vi "getProcedureList.vi"(8 "error in (no error)":errorcluster, 11 "IList in":refnum<class "IList.lvclass">) -> (0 "error out":errorcluster, 2 "devices out":refnum<class "IProcedure.lvclass">[](array[class]))   [LabVIEW 2022 SP3, in "openDAQ.lvlib" / "daqCoreTypes.lvlib" / "IList.lvclass"]
uses:
  IList.lvclass
  IProcedure/IProcedure.lvclass
  Errors/TypeDef/errorCodes.ctl
  Errors/Errors.lvclass
  IIterator/IIterator.lvclass
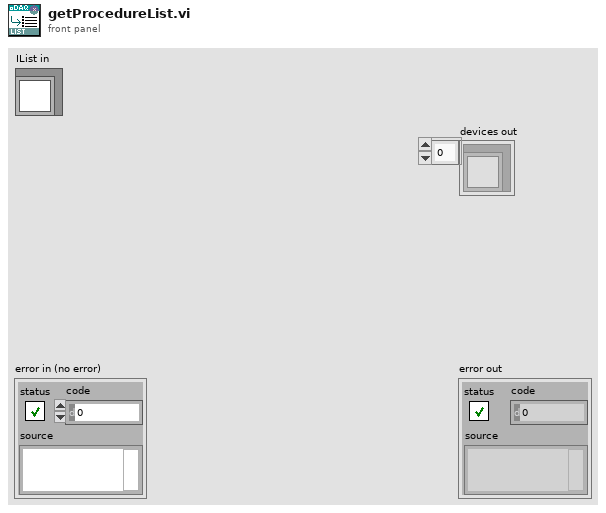
[diagram p1: front panel]
types:
  T1 = typedef "openDAQ.lvlib/daqCoreTypes.lvlib/Errors.lvclass/errorCodes.ctl" = u16
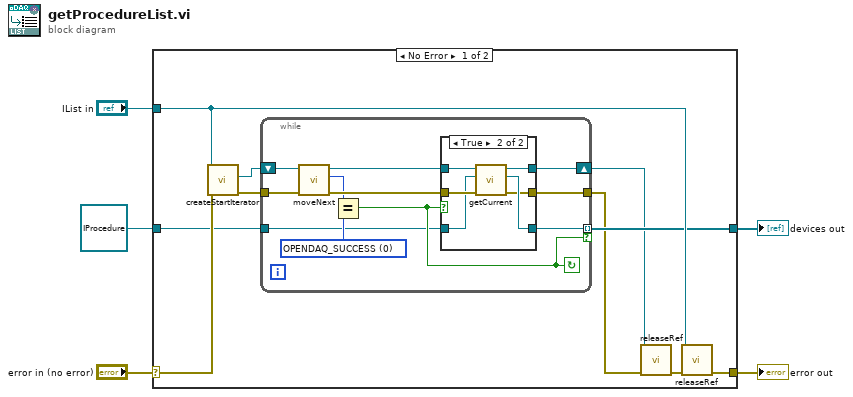
[diagram p0: block diagram]
diagram:
  n1 = case shown="No Error" "error in (no error)" {
    selector: "error in (no error)" -> [w11 w35]
    tunnel: [w15 w35] -> w4
    tunnel: "IList in" -> [w12 _]
    tunnel: refnum<class "IProcedure.lvclass"> refnum ("openDAQ.lvlib:IBaseObject.lvlib:IProcedure.lvlib:IProcedure.lvclass") -> [w6 _]
    tunnel: [w10 _] -> w2
    frame No Error {
      n2 = call "createStartIterator.vi"("error in (no error)"=w11, "IList in"=w12) -> ("error out"=w13:errorcluster, "IIterator out"=w14:refnum<class "IIterator.lvclass">)  [unwired: 7 in, 1 out]
      n3 = while {
        tunnel: w13 -> [w24]
        tunnel: [w21] -> w8
        shift-right: [w20] -> w7
        shift-left: w14 -> [w25]
        tunnel: [w17] -> w10 mode=indexing if=w19
        tunnel: w6 -> [w16]
        stop <- w19 continue-if-true
        w18 = T1 0 items=["OPENDAQ_SUCCESS"=0, "OPENDAQ_NO_MORE_ITEMS"=5] ("errorCodes")
        n4 = call "moveNext.vi"("error in (no error)"=w24, "IIterator in"=w25) -> ("error out"=w26:errorcluster, "errorCode out"=w23:T1, "IIterator out"=w22:refnum<class "IIterator.lvclass">)  [unwired: 7 in]
        n5 = Equal?(x=w23, y=w18) -> (x = y?=w19:bool)
        n6 = case shown="True" w19 {
          tunnel: w22 -> [w27 w33]
          tunnel: w26 -> [w28 w34]
          tunnel: [w28 w30] -> w21
          tunnel: [w27 w32] -> w20
          tunnel: [_ w31] -> w17
          tunnel: w16 -> [_ w29]
          frame False {
          }
          frame True {
            n7 = call "getCurrent.vi"("error in (no error)"=w34, "baseObject in"=w29, "IIterator in"=w33) -> ("error out"=w30:errorcluster, "baseObject out"=w31:refnum<class "IProcedure.lvclass">, "IIterator out"=w32:refnum<class "IIterator.lvclass">)  [unwired: 6 in]
          }
        }
      }
      n8 = call-dynamic "releaseRef.vi"("error in (no error)"=w8, "IBaseObject in"=w7) -> ("error out"=w9:errorcluster)  [unwired: 9 in]
      n9 = call-dynamic "releaseRef.vi"("error in (no error)"=w9, "IBaseObject in"=w12) -> ("error out"=w15:errorcluster)  [unwired: 9 in]
    }
    frame Error {
    }
  }
  "error out" <- w4
  "devices out" <- w2
